vi "BK Precision 8500B Series List Program.vi"() -> ()   [LabVIEW 2024]
doc: "Exemplifies creating a simple list program to run."
uses:
  BK Precision 8500B Series.lvlib
panel:
  in  "VISA resource name":refnum<visa-resource-name>
  out "V_CH":dbl caption="V_CH1" format="%#.4f"
  out "A_CH":dbl caption="V_CH1" format="%#.4f"
  out "W_CH":dbl caption="V_CH1" format="%.3f"
  in  "Number of Steps":i32=1 min=1 max=100 step=1
  in  "Mode Ext":u16[](array[ring]) caption="Mode" items=["CC", "CV", "CR", "CW"]
  in  "Level (A) Ext":dbl[](array[numeric]) caption="Level\n(A/V/W/Ohm)"
  in  "Time Ext":u32[](array[numeric]) caption="Time (s)" min=1 max=1000
  in  "Input \nState":bool[](array[boolean])
  # "(c) 2019 B&K Precision Corporation.  ALL RIGHTS RESERVED."
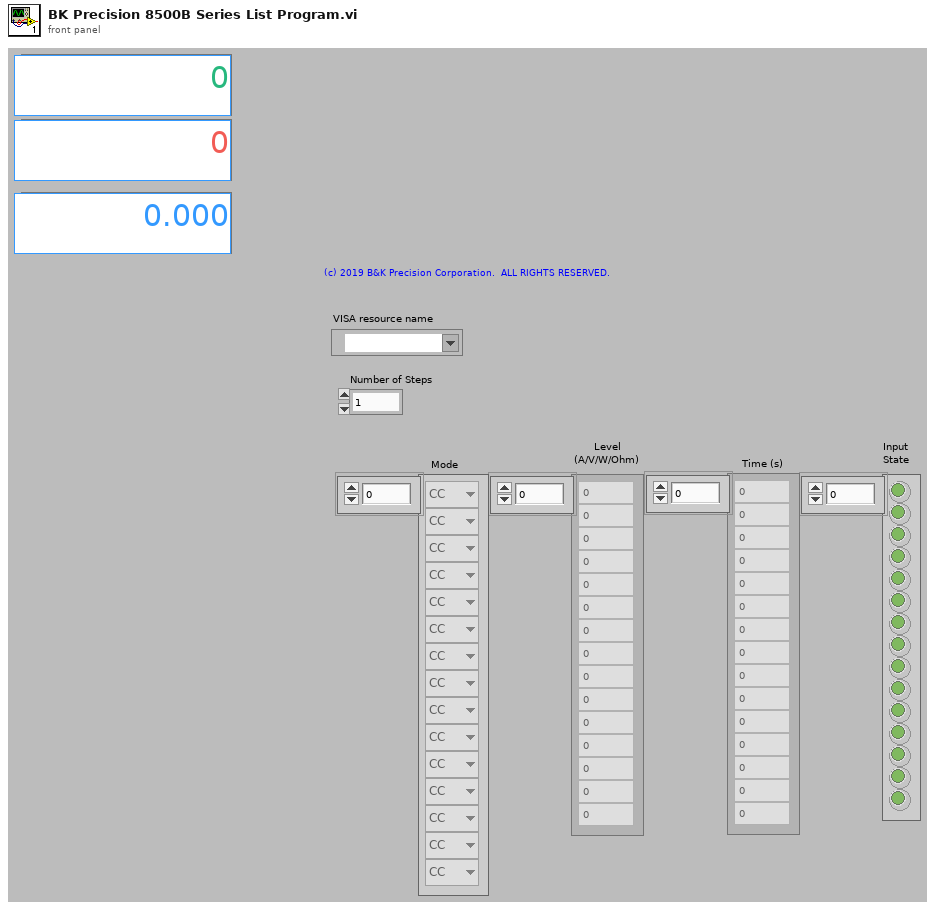
[diagram p1: front panel]
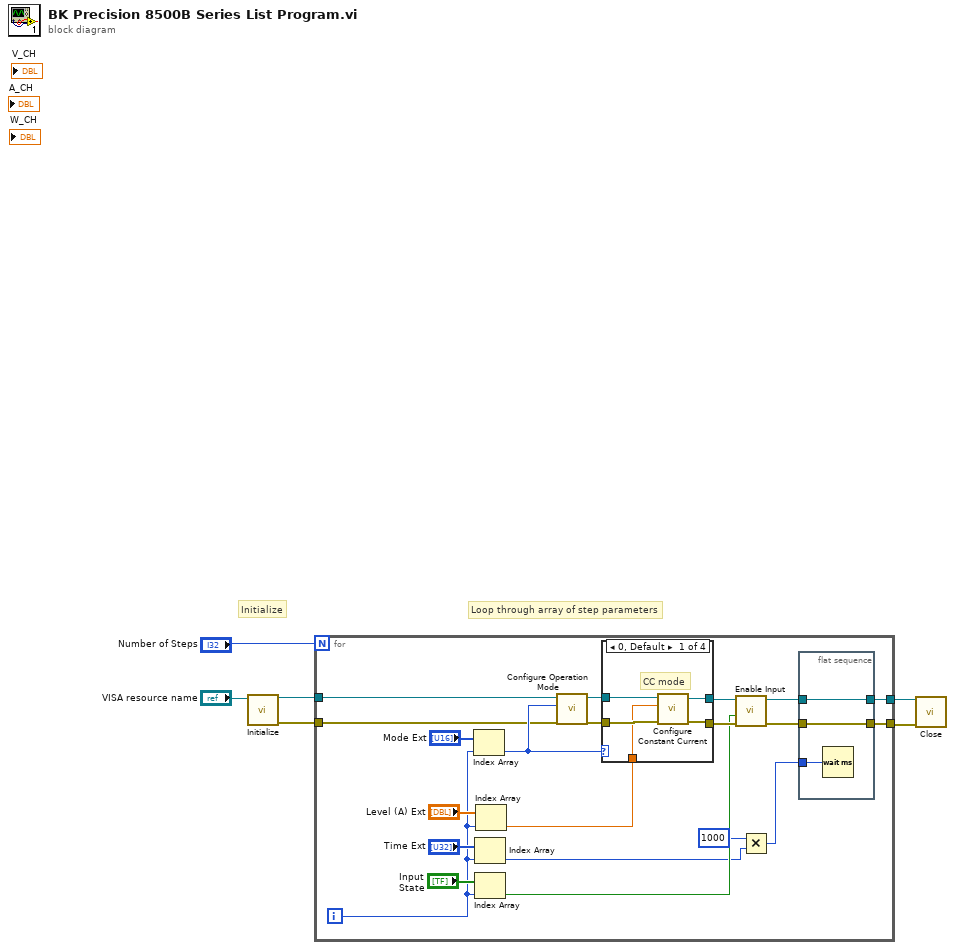
[diagram p0: block diagram]
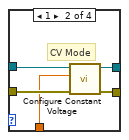
[diagram p2: hidden frame]
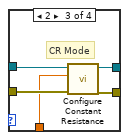
[diagram p3: hidden frame]
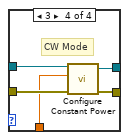
[diagram p4: hidden frame]
diagram:
  # "Loop through array of step parameters"
  # "Initialize"
  n1 = call "Initialize.vi"("VISA resource name"="VISA resource name") -> ("error out"=w4:errorcluster, "VISA resource name out"=w5:refnum<visa-resource-name>)  [unwired: 9 in]
  n2 = for {
    N: "Number of Steps" -> [_]
    tunnel: w5 -> [w14]
    tunnel: w4 -> [w13]
    tunnel: [w10] -> w1
    tunnel: [w7] -> w2
    i -> [w12]
    n3 = Index Array(array="Mode Ext", index=w12) -> (element=w23:u16)
    n4 = Index Array(array="Time Ext", index=w12) -> (element=w16:u32)
    n5 = Index Array(array="Input \nState", index=w12) -> (element=w17:bool)
    n6 = Index Array(array="Level (A) Ext", index=w12) -> (element=w20:dbl)
    n7 = call "Configure Operation Mode.vi"("error in (no error)"=w13, "Operation Mode (0:CC)"=w23, "VISA resource name"=w14) -> ("error out"=w21:errorcluster, "VISA resource name out"=w22:refnum<visa-resource-name>)  [unwired: 7 in]
    n8 = case shown="0, Default" w23 {
      tunnel: w22 -> [w35 w40 w45 w50]
      tunnel: w21 -> [w34 w39 w44 w49]
      tunnel: w20 -> [w33 w38 w43 w48]
      tunnel: [w32 w37 w42 w47] -> w19
      tunnel: [w31 w36 w41 w46] -> w18
      frame 0, Default {
        # "CC mode"
        n9 = call "Configure Constant Current.vi"("error in (no error)"=w34, "CC Current (0)"=w33, "VISA resource name"=w35) -> ("error out"=w31:errorcluster, "VISA resource name out"=w32:refnum<visa-resource-name>)  [unwired: 7 in]
      }
      frame 1 {
        # "CV Mode"
        n10 = call "Configure Constant Voltage.vi"("error in (no error)"=w39, "CV Voltage (0.1)"=w38, "VISA resource name"=w40) -> ("error out"=w36:errorcluster, "VISA resource name out"=w37:refnum<visa-resource-name>)  [unwired: 7 in]
      }
      frame 2 {
        # "CR Mode"
        n11 = call "Configure Constant Resistance.vi"("error in (no error)"=w44, "CR Resistance (1)"=w43, "VISA resource name"=w45) -> ("error out"=w41:errorcluster, "VISA resource name out"=w42:refnum<visa-resource-name>)  [unwired: 7 in]
      }
      frame 3 {
        # "CW Mode"
        n12 = call "Configure Constant Power.vi"("error in (no error)"=w49, "CW Power (1)"=w48, "VISA resource name"=w50) -> ("error out"=w46:errorcluster, "VISA resource name out"=w47:refnum<visa-resource-name>)  [unwired: 7 in]
      }
    }
    n13 = call "Enable Input.vi"("error in (no error)"=w18, "Enable Input (F: False)"=w17, "VISA resource name"=w19) -> ("error out"=w9:errorcluster, "VISA resource name out"=w8:refnum<visa-resource-name>)  [unwired: 7 in]
    n14 = Multiply(x=u32 1000, y=w16) -> (x*y=w11:u32)
    n15 = flat-sequence {
      tunnel: w11 -> [w30]
      tunnel: [w29] -> w10
      tunnel: w9 -> [w29]
      tunnel: w8 -> [w28]
      tunnel: [w28] -> w7
      frame #0 {
        n16 = Wait (ms)(milliseconds to wait=w30) -> ()  [unwired: 1 out]
      }
    }
  }
  n17 = call "Close.vi"("error in (no error)"=w1, "VISA resource name"=w2) -> ()  [unwired: 9 in, 1 out]
